vi "Temporary Password Generator.vi"() -> (3 "Temporary Password":string)   [LabVIEW 2020, in "User Configuration Manager.lvlib" / "User Configuration Manager.lvclass"]
uses:
  <vilib>/gpm_packages/@cs/user-manager/Source/User Configuration Manager/User Configuration Manager.lvclass
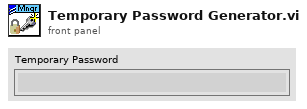
[diagram p1: front panel]
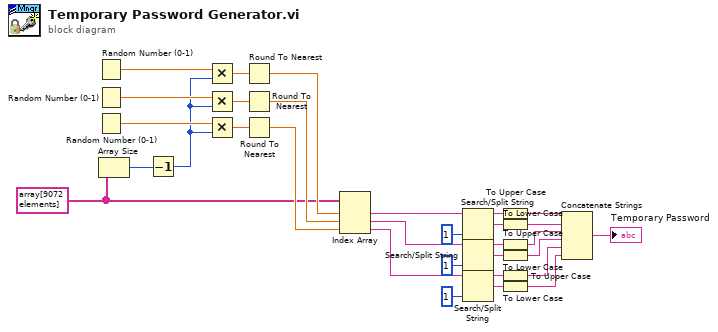
[diagram p0: block diagram]
diagram:
  w1 = string[] array[9072 elements] ("sorted array")
  n1 = Random Number (0-1)() -> (number: 0 to 1=w28:dbl)
  n2 = Random Number (0-1)() -> (number: 0 to 1=w29:dbl)
  n3 = Random Number (0-1)() -> (number: 0 to 1=w30:dbl)
  n4 = Array Size(array=w1) -> (size(s)=w31:i32)
  n5 = Decrement(x=w31) -> (x-1=w27:i32)
  n6 = Multiply(x=w28, y=w27) -> (x*y=w26:dbl)
  n7 = Multiply(x=w29, y=w27) -> (x*y=w25:dbl)
  n8 = Multiply(x=w30, y=w27) -> (x*y=w24:dbl)
  n9 = Round To Nearest(number=w26) -> (nearest integer value=w23:dbl)
  n10 = Round To Nearest(number=w25) -> (nearest integer value=w22:dbl)
  n11 = Round To Nearest(number=w24) -> (nearest integer value=w21:dbl)
  n12 = Index Array(array=w1, index #1=w23, index #2=w22, index #3=w21) -> (element #1=w15:string, element #2=w8:string, element #3=w7:string)
  n13 = Search/Split String(string=w15, offset (0)=1) -> (substring before match=w18:string, match + rest of string=w19:string)  [unwired: 1 in, 1 out]
  n14 = Search/Split String(string=w8, offset (0)=1) -> (substring before match=w14:string, match + rest of string=w13:string)  [unwired: 1 in, 1 out]
  n15 = Search/Split String(string=w7, offset (0)=1) -> (substring before match=w9:string, match + rest of string=w10:string)  [unwired: 1 in, 1 out]
  n16 = To Upper Case(1:w18) -> (0:w17:string)
  n17 = To Lower Case(string=w19) -> (all lower case string=w16:string)
  n18 = To Upper Case(1:w14) -> (0:w6:string)
  n19 = To Lower Case(string=w13) -> (all lower case string=w5:string)
  n20 = To Upper Case(1:w9) -> (0:w4:string)
  n21 = To Lower Case(string=w10) -> (all lower case string=w3:string)
  n22 = Concatenate Strings(w17, w16, w6, w5, w4, w3) -> (→"Temporary Password":string)
